vi "Nigel Tamagotchi Basic Actor Main.vi"() -> ()   [LabVIEW 2026]
uses:
  Parent Classes/Message/Message.lvclass
  Tamagotchi Basic Actor/Tamagotchi Basic Actor.lvclass
  1_QMH/Type Defs/Controls Cluster.ctl
  Messages/Update UI Message/Update UI Message.lvclass
  Messages/Update Cycles Message/Update Cycles Message.lvclass
  Messages/Feed Message/Feed Message.lvclass
  Messages/Clean Message/Clean Message.lvclass
  Messages/Sleep Message/Sleep Message.lvclass
  Messages/Spaghetti Message/Spaghetti Message.lvclass
  Messages/Broken Arrow Message/Broken Arrow Message.lvclass
  Messages/Fixed Bug Message/Fixed Bug Message.lvclass
panel:
  in  "Stop":bool
  out "Age (cycles)":u32
  out "Mood":string
  out "Cleanliness":i16(slide)=100 scale=0.0..100.0
  out "Energy":i16(slide)=100 scale=0.0..100.0
  out "Hunger":i16(slide) scale=0.0..100.0
  in  "Fixed Bug Button":bool
  in  "Broken Arrow Button":bool
  in  "Spagetti Button":bool
  in  "Sleep Button":bool
  in  "Clean Button":bool
  in  "Feed Button":bool
  out "Pict Ring":u16(ring)
  # "Nigel-gotchi (Basic Actor)"
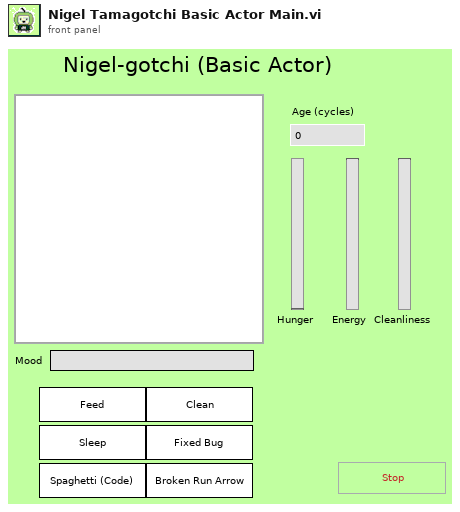
[diagram p1: front panel]
types:
  T1 = typedef "Controls Cluster.ctl" = cluster{"Pict Ring":refnum<vi>, "Mood":refnum<vi>, "Cleanliness":refnum<vi>, "Hunger":refnum<vi>, "Energy":refnum<vi>, "Age (cycles)":refnum<vi>}
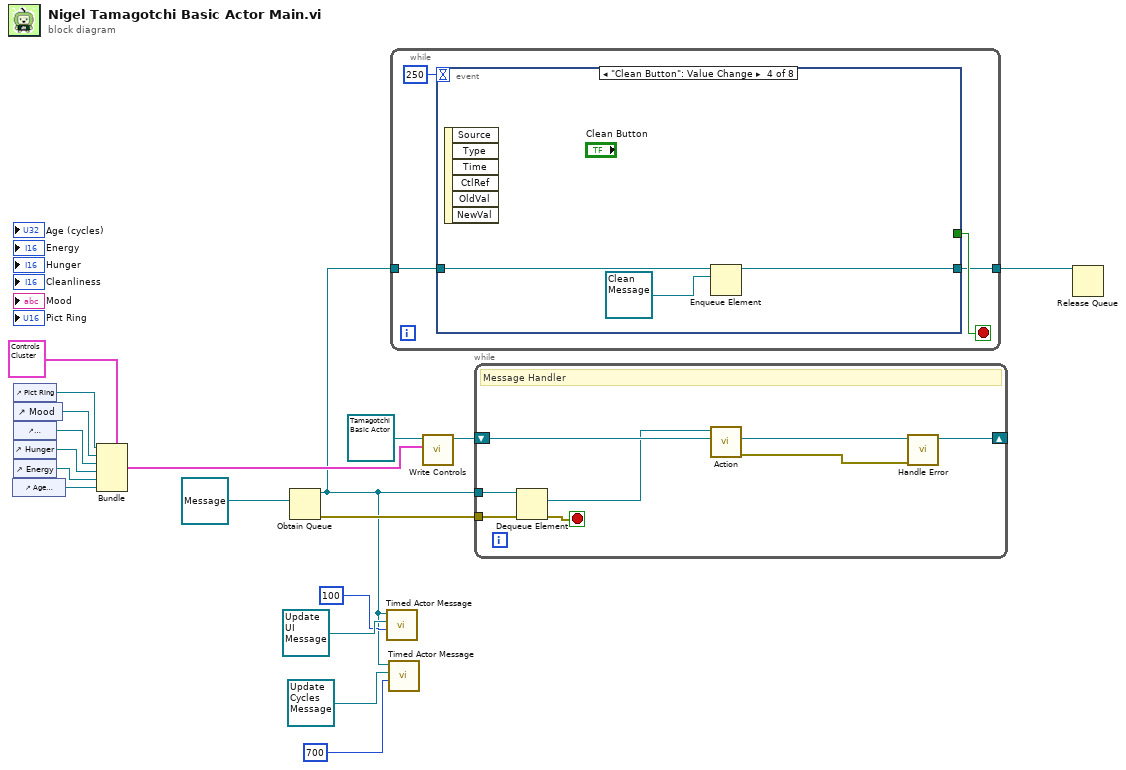
[diagram p0: block diagram]
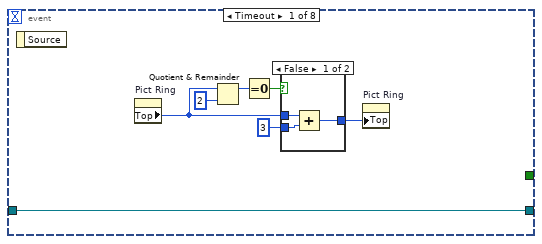
[diagram p2: hidden frame]
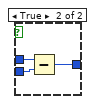
[diagram p3: hidden frame]
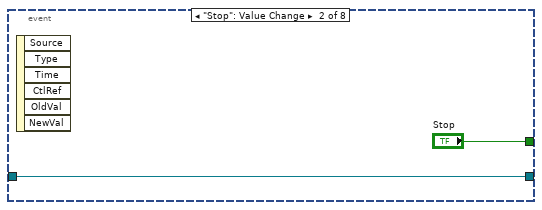
[diagram p4: hidden frame]
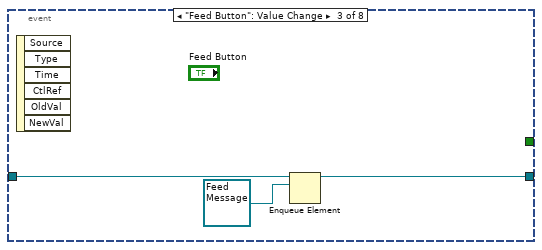
[diagram p5: hidden frame]
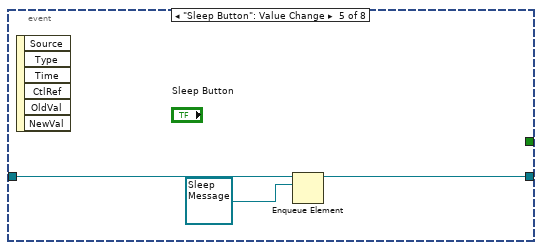
[diagram p6: hidden frame]
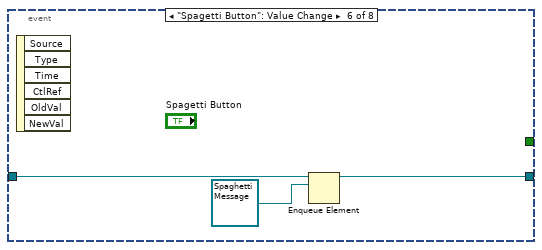
[diagram p7: hidden frame]
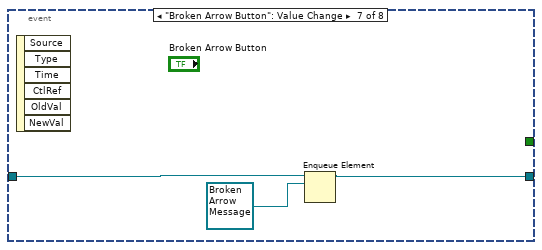
[diagram p8: hidden frame]
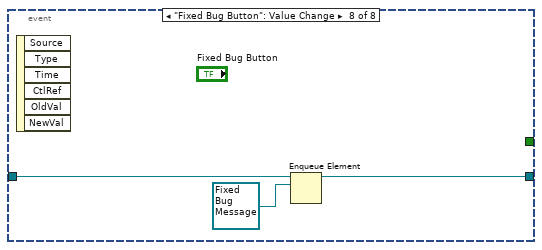
[diagram p9: hidden frame]
diagram:
  n1 = control-ref of="Age (cycles)"() -> (w10:refnum<vi>)
  n2 = control-ref of="Pict Ring"() -> (w15:refnum<vi>)
  n3 = control-ref of="Mood"() -> (w14:refnum<vi>)
  n4 = control-ref of="Cleanliness"() -> (w13:refnum<vi>)
  n5 = control-ref of="Hunger"() -> (w12:refnum<vi>)
  n6 = control-ref of="Energy"() -> (w11:refnum<vi>)
  n7 = Bundle(cluster=T1 {"Pict Ring"=refnum, "Mood"=refnum, "Cleanliness"=refnum, "Hunger"=refnum, "Energy"=refnum, "Age (cycles)"=refnum} ("Controls"), "Pict Ring"=w15, "Mood"=w14, "Cleanliness"=w13, "Hunger"=w12, "Energy"=w11, "Age (cycles)"=w10) -> (w6:T1)
  n8 = Obtain Queue(element data type=refnum<class "Message.lvclass"> refnum ("Message.lvclass")) -> (queue out=w1:refnum<queue>, error out=w18:errorcluster)  [unwired: 4 in, 1 out]
  n9 = call "Timed Actor Message.vi"("Interval (ms)"=u32 100 ("milliseconds to wait"), "Message"=refnum<class "Update UI Message.lvclass"> refnum ("Update UI Message.lvclass"), "Message Queue"=w1) -> ()  [unwired: 9 in]
  n10 = call "Timed Actor Message.vi"("Interval (ms)"=u32 700 ("milliseconds to wait"), "Message"=refnum<class "Update Cycles Message.lvclass"> refnum ("Update Cycles Message.lvclass"), "Message Queue"=w1) -> ()  [unwired: 9 in]
  n11 = while {
    tunnel: w1 -> [w21]
    tunnel: [w20] -> w17
    stop <- w22 stop-if-true
    n12 = event shown="[3] \"Clean Button\": Value Change" {
      selector: _ -> [_ _ _ _ _ _ _ _]
      dyn-events: _ -> [_ _ _ _ _ _ _ _]
      timeout: 250 -> [_ _ _ _ _ _ _ _]
      tunnel: [_ "Stop" _ _ _ _ _ _] -> w22
      tunnel: w21 -> [w29 w36 w40 w43 w46 w49 w52 w55]
      tunnel: [w29 w36 w39 w42 w45 w48 w51 w54] -> w20
      event Timeout {
        n13 = event-data() -> ()  [unwired: 1 in, 1 out]
        n14 = property on="Pict Ring" class="Ring (strict)"() -> ("Top"=w27:i32)  [unwired: 2 in, 2 out]
        n15 = Quotient & Remainder(x=w27, y=2) -> (x-y*floor(x/y)=w25:i32)  [unwired: 1 out]
        n16 = Equal To 0?(x=w25) -> (x = 0?=w26:bool)
        n17 = case shown="False" w26 {
          tunnel: w27 -> [w32 w35]
          tunnel: 3 ("y") -> [w31 w34]
          tunnel: [w30 w33] -> w28
          frame False {
            n18 = Add(x=w32, y=w31) -> (x+y=w30:i32)
          }
          frame True {
            n19 = Subtract(x=w35, y=w34) -> (x-y=w33:i32)
          }
        }
        n20 = property on="Pict Ring" class="Ring (strict)"("Top"=w28) -> ()  [unwired: 2 in, 2 out]
      }
      event "Stop": Value Change {
        n21 = event-data() -> ()  [unwired: 1 in, 6 out]
      }
      event "Feed Button": Value Change {
        n22 = event-data() -> ()  [unwired: 1 in, 6 out]
        n23 = Enqueue Element(queue=w40, element=refnum<class "Feed Message.lvclass"> refnum ("Feed Message.lvclass")) -> (queue out=w39:refnum<queue>)  [unwired: 2 in, 2 out]
      }
      event "Clean Button": Value Change {
        n24 = event-data() -> ()  [unwired: 1 in, 6 out]
        n25 = Enqueue Element(queue=w43, element=refnum<class "Clean Message.lvclass"> refnum ("Clean Message.lvclass")) -> (queue out=w42:refnum<queue>)  [unwired: 2 in, 2 out]
      }
      event "Sleep Button": Value Change {
        n26 = event-data() -> ()  [unwired: 1 in, 6 out]
        n27 = Enqueue Element(queue=w46, element=refnum<class "Sleep Message.lvclass"> refnum ("Sleep Message.lvclass")) -> (queue out=w45:refnum<queue>)  [unwired: 2 in, 2 out]
      }
      event "Spagetti Button": Value Change {
        n28 = event-data() -> ()  [unwired: 1 in, 6 out]
        n29 = Enqueue Element(queue=w49, element=refnum<class "Spaghetti Message.lvclass"> refnum ("Spaghetti Message.lvclass")) -> (queue out=w48:refnum<queue>)  [unwired: 2 in, 2 out]
      }
      event "Broken Arrow Button": Value Change {
        n30 = event-data() -> ()  [unwired: 1 in, 6 out]
        n31 = Enqueue Element(queue=w52, element=refnum<class "Broken Arrow Message.lvclass"> refnum ("Borken Arrow Message.lvclass")) -> (queue out=w51:refnum<queue>)  [unwired: 2 in, 2 out]
      }
      event "Fixed Bug Button": Value Change {
        n32 = event-data() -> ()  [unwired: 1 in, 6 out]
        n33 = Enqueue Element(queue=w55, element=refnum<class "Fixed Bug Message.lvclass"> refnum ("Fixed Bug Message.lvclass")) -> (queue out=w54:refnum<queue>)  [unwired: 2 in, 2 out]
      }
    }
  }
  n34 = call-dynamic "Write Controls.vi"("Controls"=w6, "Nigel Tamagotchi in"=refnum<class "Tamagotchi Basic Actor.lvclass"> refnum ("Nigel Tamagotchi.lvclass")) -> ("Nigel Tamagotchi out"=w7:refnum<class "Tamagotchi Basic Actor.lvclass">)  [unwired: 8 in, 1 out]
  n35 = while {
    tunnel: w1 -> [w63]
    tunnel: w18 -> [w62]
    shift-right: [w59] -> _
    shift-left: w7 -> [w58]
    stop <- w61 stop-if-true
    # "Message Handler"
    n36 = Dequeue Element(queue=w63, error in (no error)=w62) -> (element=w56:refnum<class "Message.lvclass">, error out=w61:errorcluster)  [unwired: 1 in, 2 out]
    n37 = call-dynamic "Action.vi"("Actor in"=w58, "Message in"=w56) -> ("error out"=w60:errorcluster, "Actor out"=w57:refnum<class "Tamagotchi Basic Actor.lvclass">)  [unwired: 7 in, 1 out]
    n38 = call "Handle Error.vi"("error in (no error)"=w60, "Nigel Tamagotchi in"=w57) -> ("Nigel Tamagotchi out"=w59:refnum<class "Tamagotchi Basic Actor.lvclass">)  [unwired: 8 in, 1 out]
  }
  n39 = Release Queue(queue=w17) -> ()  [unwired: 2 in, 3 out]
